vi "Init.vi"(8 "error in":errorcluster, 11 "gRPC XNET Read Raw CAN Frame Strategy in":refnum<class "gRPC XNET Read Raw CAN Frame Strategy.lvclass">) -> (0 "error out":errorcluster, 3 "gRPC XNET Read Raw CAN Frame Strategy out":refnum<class "gRPC XNET Read Raw CAN Frame Strategy.lvclass">)   [LabVIEW 2024, in "gRPC XNET Read Raw CAN Frame Strategy.lvclass"]
uses:
  gRPC XNET Read Raw CAN Frame Strategy.lvclass
  grpc-xnet/grpc-xnet_client/RPC Messages/nixnet_grpc_CreateSessionRequest_mode_enum/nixnet_grpc_CreateSessionRequest_mode_enum.lvclass
  grpc-xnet/grpc-xnet_client/RPC Messages/nixnet_grpc_CreateSessionRequest_mode_enum/nixnet_grpc_CreateSessionRequest_mode_enum.lvclass/nixnet_grpc_CreateSessionRequest_mode_enum.ctl
  gRPC XNET Read Raw CAN Frame Strategy.lvclass/gRPC XNET Read Raw CAN Frame Strategy.ctl
  Source/Interfaces/IConfiguration/IConfiguration.lvclass
  grpc-xnet/grpc-xnet_client/RPC Messages/nixnet_grpc_CreateSessionMode.ctl
  grpc-xnet/grpc-xnet_client/grpc-xnet_client.lvlib
  grpc-xnet/grpc-xnet_client/RPC Messages/nidevice_grpc_SessionInitializationBehavior.ctl
  grpc-xnet/grpc-xnet_client/RPC Messages/nixnet_grpc_CreateSessionRequest.ctl
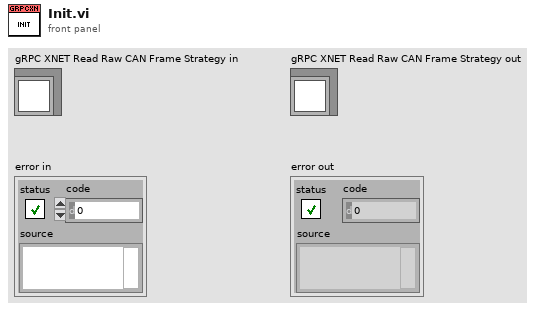
[diagram p1: front panel]
types:
  T1 = typedef "grpc-xnet_client.lvlib/nixnet_grpc_CreateSessionRequest.ctl" = cluster{"session_name":string, "database_name":string, "cluster_name":string, "list":string, "interface_name":string, "nixnet_grpc_CreateSessionRequest_mode_enum":refnum<class "nixnet_grpc_CreateSessionRequest_mode_enum.lvclass">, "initialization_behavior":T2}
  T2 = typedef "grpc-xnet_client.lvlib/nidevice_grpc_SessionInitializationBehavior.ctl" = enum32{"SESSION_INITIALIZATION_BEHAVIOR_UNSPECIFIED", "SESSION_INITIALIZATION_BEHAVIOR_INITIALIZE_NEW", "SESSION_INITIALIZATION_BEHAVIOR_ATTACH_TO_EXISTING"}
  T3 = typedef "grpc-xnet_client.lvlib/nixnet_grpc_CreateSessionMode.ctl" = enum32{"CREATE_SESSION_MODE_SIGNAL_IN_SINGLE_POINT", "CREATE_SESSION_MODE_SIGNAL_IN_WAVEFORM", "CREATE_SESSION_MODE_SIGNAL_IN_XY", "CREATE_SESSION_MODE_SIGNAL_OUT_SINGLE_POINT", "CREATE_SESSION_MODE_SIGNAL_OUT_WAVEFORM", "CREATE_SESSION_MODE_SIGNAL_OUT_XY", "CREATE_SESSION_MODE_FRAME_IN_STREAM", "CREATE_SESSION_MODE_FRAME_IN_QUEUED", "CREATE_SESSION_MODE_FRAME_IN_SINGLE_POINT", "CREATE_SESSION_MODE_FRAME_OUT_STREAM", "CREATE_SESSION_MODE_FRAME_OUT_QUEUED", "CREATE_SESSION_MODE_FRAME_OUT_SINGLE_POINT", "CREATE_SESSION_MODE_SIGNAL_CONVERSION_SINGLE_POINT"}
  T4 = typedef "grpc-lvsupport-release.lvlib/grpcId.ctl" = u64
  T5 = typedef "grpc-xnet_client.lvlib/nixnet_grpc_CreateSessionResponse.ctl" = cluster{"status":i32, "session":T6, "new_session_initialized":bool}
  T6 = typedef "grpc-xnet_client.lvlib/nidevice_grpc_Session.ctl" = cluster{"name":string}
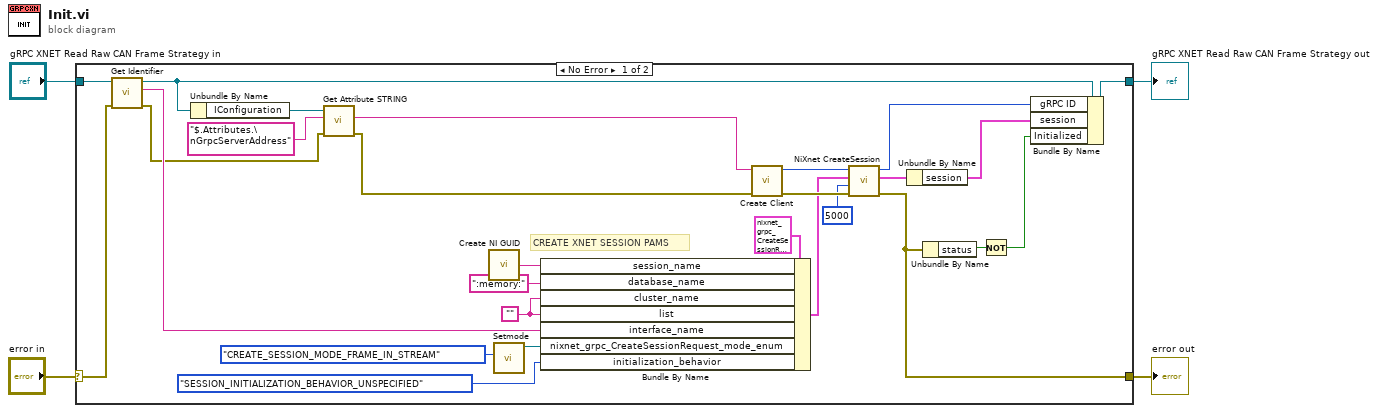
[diagram p0: block diagram]
diagram:
  n1 = case shown="No Error" "error in" {
    selector: "error in" -> [w17 w33]
    tunnel: "gRPC XNET Read Raw CAN Frame Strategy in" -> [w21 w32]
    tunnel: [w11 w32] -> w2
    tunnel: [w7 w33] -> w1
    frame No Error {
      w22 = ""
      # "CREATE XNET SESSION PAMS"
      n2 = call-dynamic "Get Identifier.vi"("error in"=w17, "gRPC XNET Read Raw CAN Frame Strategy in"=w21) -> ("error out"=w14:errorcluster, "Instrument Identifier"=w18:string, "gRPC XNET Read Raw CAN Frame Strategy out"=w19:refnum<class "gRPC XNET Read Raw CAN Frame Strategy.lvclass">)  [unwired: 7 in]
      n3 = Unbundle By Name(w19) -> ("IConfiguration"=w20:refnum<class "IConfiguration.lvclass">)
      n4 = call-dynamic "Get Attribute STRING.vi"("error in"=w14, "Attribute"="$.Attributes.\nGrpcServerAddress", "IConfiguration in"=w20) -> ("error out"=w13:errorcluster, "Value"=w12:string)  [unwired: 6 in, 1 out]
      n5 = call <vilib>:"Create NI GUID.vi"() -> ("NI GUID"=w16:string)
      n6 = call "Setmode.vi"("Set_Val"=nixnet_grpc_CreateSessionMode."CREATE_SESSION_MODE_FRAME_IN_STREAM") -> ("OneOfTemplate out"=w26:refnum<class "nixnet_grpc_CreateSessionRequest_mode_enum.lvclass">)  [unwired: 9 in, 1 out]
      n7 = Bundle By Name(cluster=T1 {"session_name"="", "database_name"="", "cluster_name"="", "list"="", "interface_name"="", "nixnet_grpc_CreateSessionRequest_mode_enum"=refnum, "initialization_behavior"=enum."SESSION_INITIALIZATION_BEHAVIOR_UNSPECIFIED"} ("Request Data"), "session_name"=w16, "database_name"=":memory:", "cluster_name"=w22, "list"=w22, "interface_name"=w18, "nixnet_grpc_CreateSessionRequest_mode_enum"=w26, "initialization_behavior"=nidevice_grpc_SessionInitializationBehavior."SESSION_INITIALIZATION_BEHAVIOR_UNSPECIFIED") -> (w24:T1)
      n8 = call "Create Client.vi"("error in"=w13, "address"=w12) -> ("error out"=w31:errorcluster, "gRPC ID Out"=w30:T4)  [unwired: 8 in]
      n9 = call "NiXnet CreateSession.vi"("error in"=w31, "timeout (ms)"=5000, "Request Data"=w24, "gRPC ID"=w30) -> ("error out"=w7:errorcluster, "Response Data"=w23:T5, "gRPC ID out"=w10:T4)  [unwired: 5 in]
      n10 = Unbundle By Name(w23) -> ("session"=w9:T6)
      n11 = Unbundle By Name(w7) -> ("status"=w6:bool)
      n12 = Not(x=w6) -> (.not. x?=w5:bool)
      n13 = Bundle By Name(cluster=w19, "gRPC ID"=w10, "session"=w9, "Initialized"=w5) -> (w11:refnum<class "gRPC XNET Read Raw CAN Frame Strategy.lvclass">)
    }
    frame Error {
    }
  }
  "error out" <- w1
  "gRPC XNET Read Raw CAN Frame Strategy out" <- w2
